vi "NI-DCPower Source DC Current for Ni-PXI4130.vi"(1 "Source Delay (Sec)":dbl=0.1 format="%_6p", 4 "Measurement:Sense":i32(ring)=1008 items=["Local"=1008, "Remote"=1009], 5 "Resource Name":string="LOAD", 6 "Channel Name":string="0", 8 "Voltage Limit":dbl=2.0 format="%_6p", 9 "Voltage Limit Range":dbl=6.0 format="%_6p", 10 "Current Level":dbl=0.1 format="%_6p", 11 "Current Level Range":dbl=0.1 format="%_6p") -> (0 "error out":errorcluster, 2 "Voltage Measurement":dbl, 3 "Current Measurement":dbl, 7 "Compliance/Limit Reached":bool)   [LabVIEW 2012]
doc: "Demonstrates how to use the DC Current Output Function to force an output current. This example initializes a session, configures the Output Function, Sense, Autorange, Current Level and Voltage Limit, initiates generation, waits for a specified delay, and measures the voltage and current output. This example uses Single Point source mode."
uses:
  <instrlib>/niDCPower/nidcpower.llb/niDCPower Source Mode.ctl
  <instrlib>/niDCPower/nidcpower.llb/niDCPower Wait For Event - Event.ctl
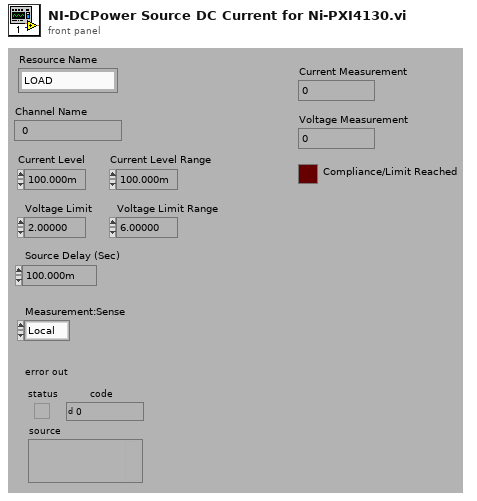
[diagram p1: front panel]
types:
  T1 = typedef "niDCPower Wait For Event - Event.ctl" = i32
  T2 = typedef "niDCPower Source Mode.ctl" = i32
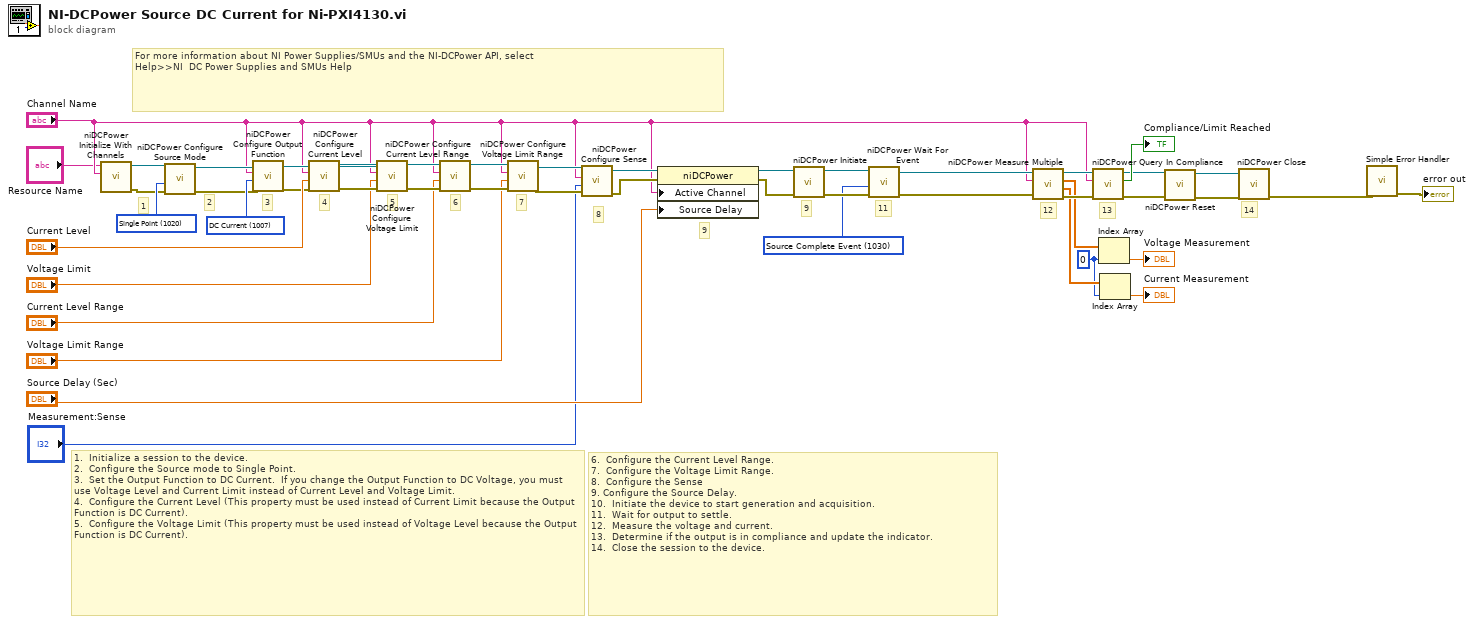
[diagram p0: block diagram]
diagram:
  w19 = T1 1030 items=["Source Complete Event"=1030, "Measure Complete Event"=1031, "Sequence Iteration Complete Event"=1032, "Sequence Engine Done Event"=1033] ("event")
  w28 = 0 ("index")
  w40 = T2 1020 items=["Single Point"=1020, "Sequence"=1021] ("source mode")
  w43 = 1007 items=["DC Voltage"=1006, "DC Current"=1007] ("output function")
  # "8"
  # "For more information about NI Power Supplies/SMUs and the NI-DCPower API, select\nHelp>>NI  DC Power Supplies and SMUs Help"
  # "9"
  # "12"
  # "11"
  # "7"
  # "6"
  # "2"
  # "1.  Initialize a session to the device.\n2.  Configure the Source mode to Single Point.\n3.  Set the Output Function to DC Current.  If you change the Output Function to DC Voltage, you must use Voltage Level and Current Limit instead of Current Level and Voltage Limit.\n4.  Configure the Current Level (This property must be used instead of Current Limit because the Output Function is DC Current).\n5.  Configure the Voltage Limit (This property must be used instead of Voltage Level because the Output Function is DC Current)."
  # "3"
  # "13"
  # "6.  Configure the Current Level Range.\n7.  Configure the Voltage Limit Range.\n8.  Configure the Sense \n9. Configure the Source Delay.\n10.  Initiate the device to start generation and acquisition.\n11.  Wait for output to settle.\n12.  Measure the voltage and current.\n13.  Determine if the output is in compliance and update the indicator.\n14.  Close the session to the device."
  # "14"
  # "9"
  # "5"
  # "4"
  # "1"
  n1 = call <instrlib>:"niDCPower Initialize With Channels.vi"("channels"="Channel Name", "resource name"="Resource Name") -> ("error out"=w15:errorcluster, "instrument handle out"=w16:refnum<k15>)  [unwired: 3 in, 5 out]
  n2 = call <instrlib>:"niDCPower Configure Source Mode.vi"("error in (no error)"=w15, "source mode"=w40, "instrument handle"=w16) -> ("error out"=w42:errorcluster, "instrument handle out"=w41:refnum<k15>)  [unwired: 7 out]
  n3 = call <instrlib>:"niDCPower Configure Output Function.vi"("error in (no error)"=w42, "output function"=w43, "channel name"="Channel Name", "instrument handle"=w41) -> ("error out"=w18:errorcluster, "instrument handle out"=w17:refnum<k15>)  [unwired: 6 out]
  n4 = call <instrlib>:"niDCPower Configure Current Level.vi"("error in (no error)"=w18, "current level"="Current Level", "channel name"="Channel Name", "instrument handle"=w17) -> ("error out"=w46:errorcluster, "instrument handle out"=w47:refnum<k15>)  [unwired: 6 out]
  n5 = call <instrlib>:"niDCPower Configure Voltage Limit.vi"("error in (no error)"=w46, "voltage limit"="Voltage Limit", "channel name"="Channel Name", "instrument handle"=w47) -> ("error out"=w39:errorcluster, "instrument handle out"=w38:refnum<k15>)  [unwired: 6 out]
  n6 = call <instrlib>:"niDCPower Configure Current Level Range.vi"("error in (no error)"=w39, "current level range"="Current Level Range", "channel name"="Channel Name", "instrument handle"=w38) -> ("error out"=w37:errorcluster, "instrument handle out"=w36:refnum<k15>)  [unwired: 6 out]
  n7 = call <instrlib>:"niDCPower Configure Voltage Limit Range.vi"("error in (no error)"=w37, "voltage limit range"="Voltage Limit Range", "channel name"="Channel Name", "instrument handle"=w36) -> ("error out"=w9:errorcluster, "instrument handle out"=w13:refnum<k15>)  [unwired: 6 out]
  n8 = call <instrlib>:"niDCPower Configure Sense.vi"("error in (no error)"=w9, "sense"="Measurement:Sense", "channel name"="Channel Name", "instrument handle"=w13) -> ("error out"=w11:errorcluster, "instrument handle out"=w12:refnum<k15>)  [unwired: 6 in]
  n9 = property class="niDCPower"(reference=w12, error in=w11, "Active Channel"="Channel Name", "Source Delay"="Source Delay (Sec)") -> (reference out=w24:refnum<k15>, error out=w25:errorcluster)
  n10 = call <instrlib>:"niDCPower Initiate.vi"("error in (no error)"=w25, "instrument handle"=w24) -> ("error out"=w20:errorcluster, "instrument handle out"=w22:refnum<k15>)  [unwired: 2 in, 6 out]
  n11 = call <instrlib>:"niDCPower Wait For Event.vi"("error in (no error)"=w20, "event"=w19, "instrument handle"=w22) -> ("error out"=w2:errorcluster, "instrument handle out"=w21:refnum<k15>)  [unwired: 1 in, 6 out]
  n12 = call <instrlib>:"niDCPower Measure Multiple.vi"("error in (no error)"=w2, "channel name"="Channel Name", "instrument handle"=w21) -> ("error out"=w32:errorcluster, "current measurements"=w29:dbl[], "voltage measurements"=w30:dbl[], "instrument handle out"=w33:refnum<k15>)  [unwired: 5 out]
  n13 = call <instrlib>:"niDCPower Query In Compliance.vi"("error in (no error)"=w32, "channel name"="Channel Name", "instrument handle"=w33) -> ("error out"=w4:errorcluster, "in compliance?"=→"Compliance/Limit Reached":bool, "instrument handle out"=w6:refnum<k15>)  [unwired: 6 out]
  n14 = Index Array(array=w30, index=w28) -> (element=→"Voltage Measurement":dbl)
  n15 = Index Array(array=w29, index=w28) -> (element=→"Current Measurement":dbl)
  n16 = call <instrlib>:"niDCPower Reset.vi"("error in (no error)"=w4, "instrument handle"=w6) -> ("error out"=w3:errorcluster, "instrument handle out"=w5:refnum<k15>)  [unwired: 8 in]
  n17 = call <instrlib>:"niDCPower Close.vi"("error in (no error)"=w3, "instrument handle"=w5) -> ("error out"=w14:errorcluster)  [unwired: 9 out]
  n18 = call <vilib>:"Simple Error Handler.vi"("error in (no error)"=w14) -> ("error out"=→"error out":errorcluster)  [unwired: 1 in, 7 out]
